vi "Dashboard Main.vi"() -> ()   [LabVIEW 2019]
uses:
  <vilib>/Utility/miscctls.llb/LVRowAndColumnTypeDef.ctl
  <vilib>/event_ctls.llb/eventvkey.ctl
  <vilib>/Rock Robotics/Network Tables/NT Read Numeric Array.vi
  <vilib>/Rock Robotics/Network Tables/NT Read Boolean.vi
  <vilib>/Rock Robotics/WPI/Dashboard/WPI_DashboardLogging Global.vi
panel:
  in  "Camera Settings Right":T1={"Frame Rate"=30, "Compression"=30, "Size"=1, "DB Camera Config"=FALSE} {"Frame Rate" scale=1.0..30.0; "Compression" scale=100.0..-1.0; "Size" items=["640x480", "320x240", "160x120"]}
  in  "Camera Name Right":string(combo)="No Camera Selection"
  out "Camera Perf":string
  in  "Camera Settings":T1={"Frame Rate"=30, "Compression"=30, "Size"=1, "DB Camera Config"=FALSE} {"Frame Rate" scale=1.0..30.0; "Compression" scale=100.0..-1.0; "Size" items=["640x480", "320x240", "160x120"]}
  in  "TCP":refnum<k5>
  in  "Rec Mode":enum32{"Stop", "Record", "Playback"}(radio)
  out "Robot IP":string
  out "Image Message":string="Timeout in Camera Communications"
  in  "Dashboard Tab":T2(tab)=enum."Custom"
  in  "Select Auto":string(combo)="Select Autonomous ..."
  out "NT Connection":bool
  out "MotorChart R":cluster{"Numeric":dbl, "Numeric":dbl}(graph)
  out "MotorChart L":cluster{"Numeric":dbl, "Numeric":dbl}(graph)
  out "MotorSliders R":cluster{"MotorSlide1":dbl, "MotorSlide2":dbl} {"MotorSlide2" scale=-1.0..1.0 scale format="%#_2e"; "MotorSlide1" scale=-1.0..1.0 scale format="%#_2e"}
  out "MotorSliders L":cluster{"MotorSlide1":dbl, "MotorSlide2":dbl} {"MotorSlide2" scale=-1.0..1.0 scale format="%#_2e"; "MotorSlide1" scale=-1.0..1.0 scale format="%#_2e"}
  out "Gyro":dbl(knob) scale=0.0..360.0
  out "JS1 Z":dbl(slide) scale=-1.0..1.0 scale format="%#_2e"
  out "JS1 Graph":cluster{"X":dbl, "Y":dbl}[](graph)
  out "JS1 Buttons":T3
  out "JS2 Z":dbl(slide) scale=-1.0..1.0 scale format="%#_2e"
  out "JS2 Graph":cluster{"X":dbl, "Y":dbl}[](graph)
  out "JS2 Buttons":T3
  out "Mode":T4(ring)=enum."Auto Disabled"
  out "Right Camera Perf":cluster{"Bandwidth (Mbps)":dbl, "FPS":dbl}
  out "Camera Image Right":T5(plugin-control)
  in  "DB/String 9":string
  in  "DB/String 8":string
  in  "DB/String 7":string
  in  "DB/String 6":string
  in  "DB/String 5":string
  in  "DB/String 4":string
  in  "DB/String 3":string
  in  "DB/String 2":string
  in  "DB/String 1":string
  in  "DB/String 0":string
  in  "DB/Slider 0":dbl(slide) scale=0.0..5.0
  in  "DB/Slider 1":dbl(slide) scale=0.0..5.0
  in  "DB/Slider 2":dbl(slide) scale=0.0..5.0
  in  "DB/Slider 3":dbl(slide) scale=0.0..5.0
  out "DB/LED 3":bool
  out "DB/LED 2":bool
  out "DB/LED 1":bool
  out "DB/LED 0":bool
  in  "DB/Button 3":bool
  in  "DB/Button 2":bool
  in  "DB/Button 1":bool
  in  "DB/Button 0":bool caption="New Name"
  out "RET BOOL":bool
  in  "RETICLE":bool caption="RET SHAPE"
  in  "Color":u32(colorbox)=16775210
  out "Intake rotation":dbl(knob) scale=-100.0..100.0
  out "version_note":string
  in  "FIRE PULSE":dbl=0.4 caption="PULSE (s)" min=0.1 max=1.0 step=0.05 format="%#.1g"
  in  "FIRE SPD":dbl=0.4 min=0.4 max=1.0 step=0.1 format="%#.1g"
  out "GAME COLOR":u32(colorbox)
  out "SENSOR COLOR":u32(colorbox)
  out "DRIVER Z":dbl
  out "DRIVER Y":dbl
  out "SHOOTER HT":dbl[](array[slide]) caption="SHOOTER Ht & Spd" scale=0.2..1.0
  out "CW ROTATION":bool
  out "CW DEPLOY":bool
  out "LIFT LOCK":bool
  out "INV DRIVE":bool
  out "FORZA":bool
  out "1 Joystick":bool
  out "NEO MOTOR TEMPS":dbl[](array[slide])=[106.99300699300699] scale=50.0..200.0
  in  "HEIGHT":i32=20
  in  "TOP":i32=130
  in  "WIDE":i32=40
  in  "LEFT":i32=140
  in  "Test Slider":dbl(slide) scale=0.0..100.0 scale format="%#_3g"
  in  "On/Off":bool caption="Solenoid"
  in  "Test Name":u16(ring) items=["Select the test to run..."]
  in  "Test Tree":string(tree)
  in  "Motor":cluster{"Value":dbl, "Enable":bool} {"Value" scale=-1.0..1.0 scale format="%#_3g"}
  out "Progress":T6 {"Test Progress" scale=0.0..100.0}
  in  "Rev/Fwd":cluster{"Forward":bool, "Reverse":bool}
  in  "Test Ring":u16(ring) items=["Monochrome", "Color"]
  out "Cmd Status":string
  in  "Execute Command":bool
  in  "Command Params":string[][](table)
  in  "Command Selection":i32(listbox)
  in  "CheckList":i32(listbox)
  out "Tree":string(tree)
  out "Camera Image":T5(plugin-control)
  out "Background":bool
  in  "Camera Name":string(combo)="No Camera Selection"
  # "HW"
  # "HW"
  # "Joysticks"
  # "Drive Motors"
  # "Front"
  # "Right"
  # "Left"
  # "Back"
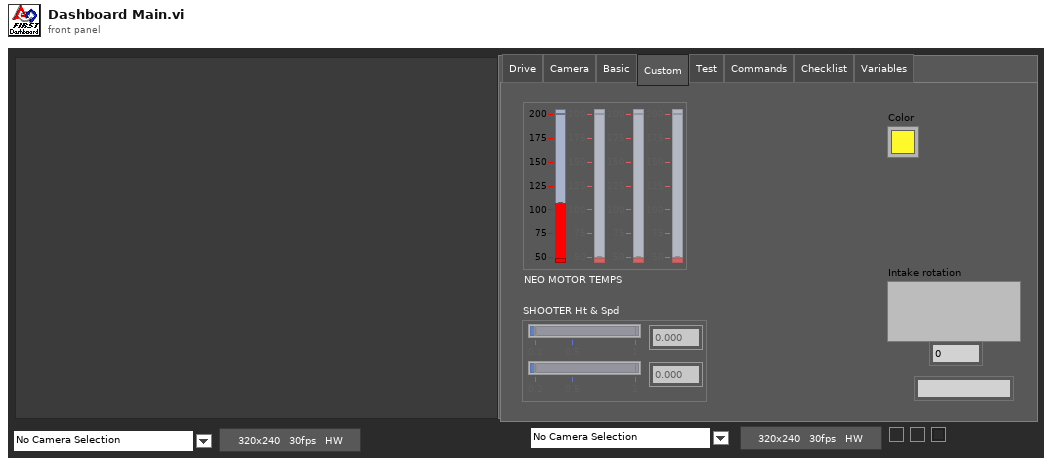
[diagram p1: front panel]
types:
  T1 = cluster{"Frame Rate":i32, "Compression":i32, "Size":u16, "DB Camera Config":bool}
  T2 = enum32{"Drive", "Camera", "Basic", "Custom", "Test", "Commands", "Checklist", "Variables"}
  T3 = cluster{bool, bool, bool, bool, bool, bool, bool, bool, bool, bool, bool, bool}
  T4 = enum8{"Tele-Op Disabled", "Tele-Op Enabled", "Auto Disabled", "Auto Enabled", "Test Disabled", "Test Enabled", "Disconnected", "No Code", "E-Stop"}
  T5 = typedef "IMAQ Image.ctl" = refnum<image>
  T6 = cluster{"Test Progress":u8, "Test Progress Text":string}
  T7 = cluster{"Save Path":path, "Interval (s)":dbl, "Keep":i32}
  T8 = typedef "Image Type" = u32
  T9 = cluster{"IDs":cluster{"RPC field ID":u16, "Unique ID":u16}, "String":string}
  T10 = cluster{"Error Strings":string, "Disable Counts":cluster{u16, u16}, "Rail Faults":cluster{u16, u16, u16}, "Robot IP":string, "DB Mode":u8, "Event Info":cluster{"Name":string, "Type":u8, "Number":u16, "Replay":u8}}
  T11 = cluster{"Storage":cluster{"Disk Free":u64, "RAM Block":u32, "RAM free":u32}, "CPU Utilization":cluster{"CPU % ISR":sgl, "CPU % Time Crit":sgl, "CPU % Timed Str":sgl, "CPU % High":sgl, "CPU % Above":sgl, "CPU % Normal":sgl, "CPU % Low":sgl}, "CAN":cluster{"% Bus Utilization":sgl, "Bus Off Cnt":u32, "TX_FIFO Full Cnt":u32, "Receive Error Cnt":u8, "Transmit Error Cnt":u8}, "HID":cluster{"HID Outputs":u32, "Rumble Low":u16, "Rumble High":u16}[]}
  T12 = cluster{"Status bits":cluster{"Test Mode":bool, "Autonomous":bool, "Enabled":bool, "Code Start":bool, "Brownout":bool, "Reserved 2":bool, "Reserved 3":bool, "E-Stop":bool}, "Code Trace":cluster{"Disabled":bool, "TeleOp":bool, "Auto":bool, "Test":bool}, "Controller Type":enum16{"unknown", "cRIO", "roboRio"}, "Code?":enum16{"unknown", "noCode", "code"}, "Battery V":dbl}
  T13 = cluster{"Control Bits":cluster{"TestMode":bool, "Autonomous":bool, "Enabled":bool, "FMS Present":bool, bool, bool, bool, "E-Stop":bool}, "Team Station ":u8, "Countdown":sgl, "Joystick Values":cluster{"Axes":dbl[], "Buttons":bool[], "POVs":i16[]}[]}
  T14 = cluster{"Axes":dbl[], "Buttons":bool[], "POVs":i16[]}[]
  T15 = cluster{"Axes":dbl[], "Buttons":bool[], "POVs":i16[]}
  T16 = cluster{"Buttons[0]":bool, "Buttons[1]":bool, "Buttons[2]":bool, "Buttons[3]":bool, "Buttons[4]":bool, "Buttons[5]":bool, "Buttons[6]":bool, "Buttons[7]":bool, "Buttons[8]":bool, "Buttons[9]":bool, "Buttons[10]":bool, "Buttons[11]":bool}
  T17 = cluster{"Camera Image":refnum<vi>, "Dashboard Tab":refnum<vi>, "Background":refnum<vi>, "Rec Mode":refnum<vi>, "Test Slider":refnum<vi>, "On/Off ":refnum<vi>, "Test Ring":refnum<vi>, "Rev/Fwd":refnum<vi>, "Test Name":refnum<vi>, "Motor":refnum<vi>, "Progress":refnum<vi>, "CheckList":refnum<vi>, "Tree":refnum<vi>, "Test Tree":refnum<vi>, "Command Params":refnum<vi>, "Command Selection":refnum<vi>, "Execute Command":refnum<vi>, "Cmd Status":refnum<vi>, "Camera Settings":refnum<vi>, "Camera Name":refnum<vi>, "Camera Perf":refnum<vi>, "Camera Settings Right":refnum<vi>, "Camera Name Right":refnum<vi>, "Camera Image Right":refnum<vi>}
  T18 = cluster{"Global Rectangle":i32[], "Contours":cluster{"Contour Type":u32, "ROI Type":u32, "Points":i32[]}[]}
  T19 = cluster{"Left":i32, "Top":i32, "Right":i32, "Bottom":i32}
  T20 = cluster{"Camera Name":string, string, "Saved DB Images Info":cluster{"Save Path":path, "Interval (s)":dbl, "Keep":i32}}
  T21 = cluster{"Camera Name Right":string, string, "Saved DB Images Info":cluster{"Save Path":path, "Interval (s)":dbl, "Keep":i32}}
  T22 = cluster{"Operation":enum16{"Update", "Clear"}, "Color Box":u32}[]
  T23 = typedef "eventvkey.ctl" = enum16{"ASCII", "Enter", "Return", "Shift", "Ctrl", "Alt", "Cmd", "Opt", "Caps", "NumLock", "Clear", "Break", "Up", "Down", "Left", "Right", "Insert", "Delete", "Home", "End", "PageUp", "PageDown", "Escape", "Help", "Pause", "ScrollLock", "F1", "F2", "F3", "F4", "F5", "F6", "F7", "F8", "F9", "F10", "F11", "F12", "F13", "F14", "F15", "F16", "F17", "F18", "F19", "F20", "F21", "F22", "F23", "F24", "Play", "VolumeUp", "VolumeDown", "Mute", "Two Byte Char"}
  T24 = cluster{"Image Size":bool, "Image Type":bool, "Pixel Value":bool, "ROI Information":bool, "Zoom Factor":bool}
  T25 = cluster{"Operation":enum16{"Update", "Clear"}, "Color Box":u32}
  T26 = typedef "LVRowAndColumnTypeDef.ctl" = cluster{"Row":i32, "Column":i32}
  T27 = cluster{"Shift":bool, "Ctrl":bool, "Alt":bool, "Cmd":bool, "Opt":bool}
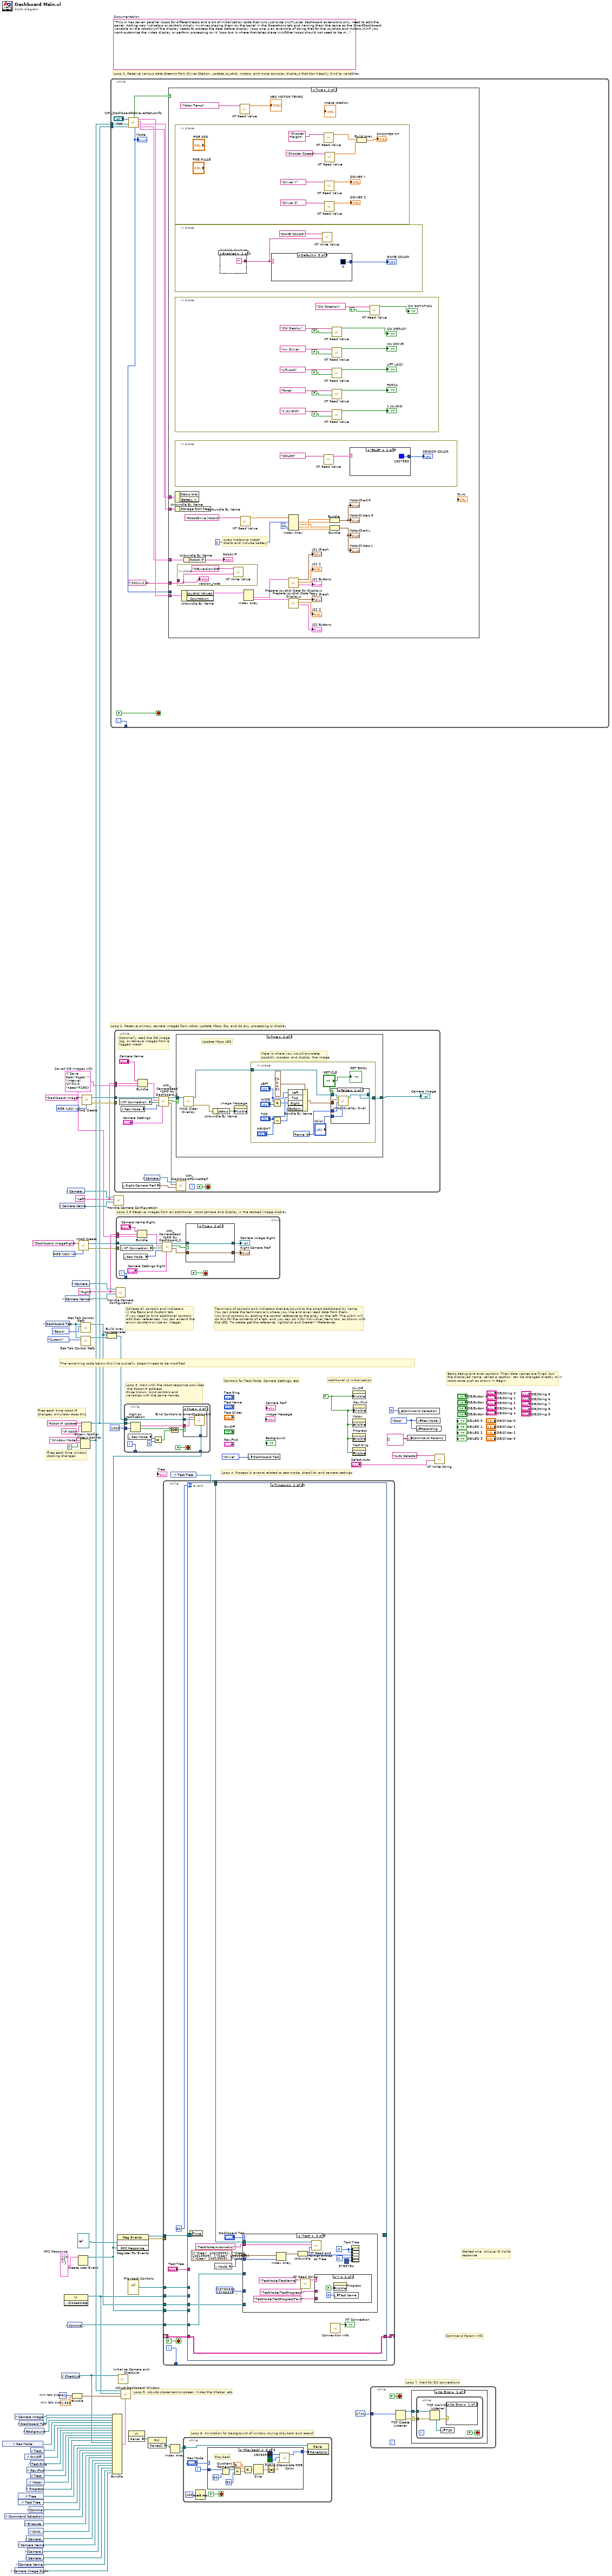
[diagram p0: block diagram]
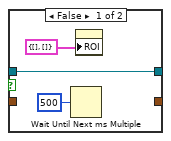
[diagram p2: hidden frame]
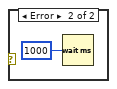
[diagram p3: hidden frame]
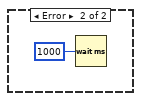
[diagram p4: hidden frame]
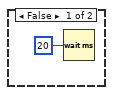
[diagram p5: hidden frame]
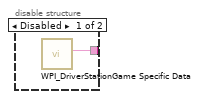
[diagram p6: hidden frame]
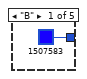
[diagram p7: hidden frame]
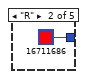
[diagram p8: hidden frame]
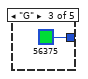
[diagram p9: hidden frame]
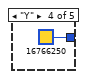
[diagram p10: hidden frame]
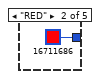
[diagram p11: hidden frame]
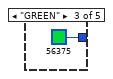
[diagram p12: hidden frame]
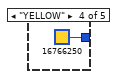
[diagram p13: hidden frame]
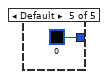
[diagram p14: hidden frame]
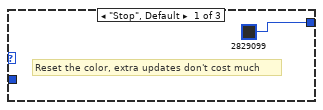
[diagram p15: hidden frame]
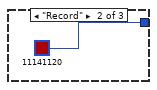
[diagram p16: hidden frame]
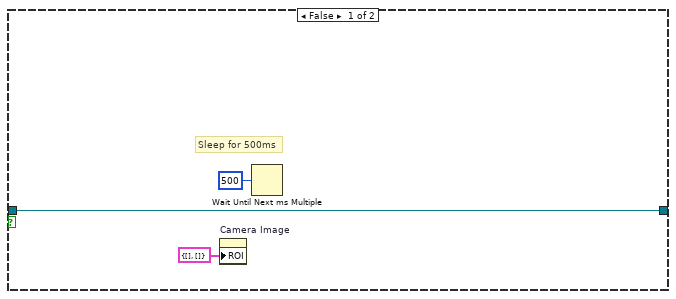
[diagram p18: hidden frame]
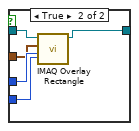
[diagram p19: hidden frame]
diagram:
  w3 = T7 {"Save Path"=path "", "Interval (s)"=1.0, "Keep"=180}  # Saved DB Images Info
  w2 = "Right"
  w1 = "Left"
  w13 = T8 4 items=["Grayscale (U8)", "Grayscale (I16)", "Grayscale (SGL)", "Complex (CSG)", "RGB (U32)", "HSL (U32)", "RGB (U64)"] ("Image Type")
  w29 = T9 {"IDs"={"RPC field ID"=0, "Unique ID"=0}, "String"=""}  # RPC Response
  w52 = 491  # min tab size
  w51 = 1.333  # min tab size
  w59 = enum32{"Stop", "Record", "Playback"}."Stop" ("Rec Mode")
  w36 = FALSE ("Visible")
  (unwired) "This VI has seven parallel loops for different tasks and a bit of initialization code that runs just once.\n\nTypical dashboard extensions only need to edit the panel. Adding new indicators or controls simply involves placing them on the panel in the Operations tab and naming them the same as the SmartDashboard variable on the robot\n\nIf the display needs to process the data before display, loop one is an example of doing that for the joysticks and motors.\n\nIf you want customize the video display or perform processing on it, loop two is where that takes place.\n\nOther loops should not need to be modified. They are pretty standard, and document the task they perform."  # Documentation
  w76 = T8 4 items=["Grayscale (U8)", "Grayscale (I16)", "Grayscale (SGL)", "Complex (CSG)", "RGB (U32)", "HSL (U32)", "RGB (U64)"] ("Image Type")
  # "Loop 2.5 Receive images from an additional  robot camera and display in the tabbed image display"
  # "Command Param Info"
  # "Started one, Unique ID holds\nresponse"
  # "Loop 7. Wait for DS connections"
  # "Basic debug and auto controls: Their data names are fixed, but\nthe displayed name, called a caption, can be changed directly or in\nrobot code such as shown in Begin."
  # "Controls for Test Mode, Camera Settings, etc."
  # "Additional UI Initialization"
  # "Loop 6. Animation for background of window during playback and record"
  # "Fires each time robot IP\nchanges, simulator does this"
  # "Fires each time window\ndocking changes."
  # "Collects all controls and indicators\nin the Basic and Custom tab.\nIf you need to bind additional controls,\nadd their references. You can extend the\nenum constant or use an integer."
  # "The remaining code below this line typically doesn't need to be modified."
  # "Loop 4. Process UI events related to test mode, checklist, and camera settings"
  # "Terminals of controls and indicators that are bound to the smart dashboard by name.\nYou can place the terminals anywhere you like and even read data from them.\nYou bind controls by adding the control reference to the array on the left. The subVI will\ndo this for the contents of a tab, and you can do it for individual items too, as shown with\nthe LED. To create get the reference, right-click and Create>>Reference."
  # "Loop 3. Wait until the robot response provides\n the Robot IP address.\nOnce known, bind controls and\nvariables with the same names."
  # "Loop 5. Adjusts placement onscreen, hides the titlebar, etc."
  # "Loop 1. Receive various data streams from Driver Station, update joystick, motors, and more complex displays that don't easily bind to variables."
  # "Loop 2. Receive primary camera images from robot, update Mbps, fps, and do any processing or display"
  n1 = control-ref of="Rec Mode"() -> (w42:refnum<vi>)
  n2 = control-ref of="Command Selection"() -> (w28:refnum<vi>)
  n3 = control-ref of="Camera Image Right"() -> (w6:refnum<vi>)
  n4 = control-ref of="Camera Image"() -> (w54:refnum<vi>)
  n5 = control-ref of="Tree"() -> (w46:refnum<vi>)
  n6 = control-ref of="Test Tree"() -> (w45:refnum<vi>)
  n7 = control-ref of="Camera Name"() -> (w19:refnum<vi>)
  n8 = control-ref of="Camera Name Right"() -> (w7:refnum<vi>)
  n9 = control-ref of="Dashboard Tab"() -> (w53:refnum<vi>)
  n10 = control-ref of="Execute Command"() -> (w30:refnum<vi>)
  n11 = control-ref of="Background"() -> (w49:refnum<vi>)
  n12 = control-ref of="On/Off"() -> (w40:refnum<vi>)
  n13 = control-ref of="Progress"() -> (w37:refnum<vi>)
  n14 = control-ref of="Camera Settings"() -> (w20:refnum<vi>)
  n15 = control-ref of="Camera Settings Right"() -> (w8:refnum<vi>)
  n16 = control-ref of="Rev/Fwd"() -> (w38:refnum<vi>)
  n17 = control-ref of="Motor"() -> (w43:refnum<vi>)
  n18 = control-ref of="Camera Perf"() -> (w18:refnum<vi>)
  n19 = control-ref of="Cmd Status"() -> (w24:refnum<vi>)
  n20 = control-ref of="Command Params"() -> (w31:refnum<vi>)
  n21 = control-ref of="Test Slider"() -> (w41:refnum<vi>)
  n22 = control-ref of="Test Ring"() -> (w39:refnum<vi>)
  n23 = control-ref of="Test Name"() -> (w44:refnum<vi>)
  n24 = control-ref of="Dashboard Tab"() -> (w57:refnum<vi>)
  n25 = control-ref of="Camera Name"() -> (w21:refnum<vi>)
  n26 = control-ref of="CheckList"() -> (w47:refnum<vi>)
  n27 = property class="VI" props=["Front Panel.Closeable"]() -> (reference out=w58:refnum<vi>)  [unwired: 2 in, 2 out]
  n28 = control-ref of="Camera Name Right"() -> (w9:refnum<vi>)
  n29 = control-ref of="Camera Settings"() -> (w22:refnum<vi>)
  n30 = control-ref of="Command Params"() -> (w23:refnum<vi>)
  n31 = control-ref of="Camera Settings Right"() -> (w10:refnum<vi>)
  n32 = Bundle("min tab size"=w52, "min tab size"=w51) -> (w50:cluster{"min tab size":i32, "min tab size":dbl})  [unwired: 1 in]
  n33 = Create User Event(user event datatype=w29) -> (user event=w25:refnum<user-event>)  [unwired: 1 in, 1 out]
  n34 = call "IMAQ Create"("Image Name"="Dashboard ImageRight", "Image Type"=w13) -> ("New Image"=w12:T5, "error out"=w11:errorcluster)  [unwired: 2 in, 1 out]
  n35 = Obtain Notifier(name (unnamed)="Window Mode", notification data type=TRUE) -> (notifier out=w34:refnum<notifier>)  [unwired: 2 in, 2 out]
  n36 = call <vilib>:"Get Tab Control Refs.vi"("Page Index"=T2."Basic" ("Dashboard Tab"), "TabControl in"=w57) -> ("ControlsOnPage"=w17:refnum<vi>[])  [unwired: 9 in]
  n37 = call <vilib>:"Get Tab Control Refs.vi"("Page Index"=T2."Custom" ("Dashboard Tab"), "TabControl in"=w57) -> ("ControlsOnPage"=w56:refnum<vi>[])  [unwired: 9 in]
  n38 = Obtain Notifier(name (unnamed)="Robot IP Update", notification data type="IP Addr" ("name (unnamed)")) -> (notifier out=w35:refnum<notifier>)  [unwired: 2 in, 2 out]
  n39 = call "IMAQ Create"("Image Name"="Dashboard Image", "Image Type"=w76) -> ("New Image"=w74:T5, "error out"=w73:errorcluster)  [unwired: 2 in, 1 out]
  n40 = Build Array (concatenate)(w17, w56) -> (w55:refnum<vi>[])
  n41 = while {
    tunnel: [w87] -> _
    tunnel: w35 -> [w81]
    tunnel: w34 -> [w78]
    i -> [w87]
    stop <- FALSE stop-if-true
    n42 = call <vilib>:"WPI_DashboardRetrieveStatusInfo.vi"("Binding Refnum"=w81, "Window Mode Notifier"=w78, "TCP Cnx"="TCP") -> ("Power and Errors"=w82:T10, "Robot Metrics"=w85:T11, "Status Info"=w86:T12, "Control Info"=w83:T13, "Robot Mode"=w80:T4, "Process?"=w84:bool)  [unwired: 3 in]
    "Mode" <- w80
    n43 = case shown="True" w84 {
      tunnel: w86 -> [_ w116]
      tunnel: w85 -> [_ w115]
      tunnel: w83 -> [_ w114]
      tunnel: w82 -> [_ w113]
      tunnel: w80 -> [_ _]
      tunnel: "2021v2.0" ("version_note") -> [_ w92]
      frame False {
        n44 = Wait (ms)(milliseconds to wait=u32 20) -> ()  [unwired: 1 out]
      }
      frame True {
        # "swap motors to match\ncharts and include battery"
        n45 = in-place {
          n46 = call-poly <vilib>:"NT Read Value.vi"("Name"="Shooter Height") -> ("Numeric"=w140:dbl)  [unwired: 9 in, 1 out]
          n47 = call-poly <vilib>:"NT Read Value.vi"("Name"="Driver Y") -> ("Numeric"=→"DRIVER Y":dbl)  [unwired: 9 in, 1 out]
          n48 = call-poly <vilib>:"NT Read Value.vi"("Name"="Driver Z") -> ("Numeric"=→"DRIVER Z":dbl)  [unwired: 9 in, 1 out]
          n49 = call-poly <vilib>:"NT Read Value.vi"("Name"="Shooter Speed") -> ("Numeric"=w138:dbl)  [unwired: 9 in, 1 out]
          n50 = Build Array(w140, w138) -> (→"SHOOTER HT":dbl[])
        }
        n51 = in-place {
          n52 = disable-structure shown="Enabled" {
            disable-tunnel: [w122 "" ("Game Specific Data")] -> w119
            frame Disabled {
              n53 = call <vilib>:"WPI_DriverStationGame Specific Data.vi"() -> ("Game Specific Data"=w122:string)  [unwired: 11 in]
            }
            frame Enabled {
            }
          }
          n54 = case shown="Default" w119 {
            tunnel: [u32 1507583 ("SENSOR COLOR") u32 16711686 ("SENSOR COLOR") u32 56375 ("SENSOR COLOR") u32 16766250 ("SENSOR COLOR") u32 0 ("SENSOR COLOR")] -> w121
            frame "B" {
            }
            frame "R" {
            }
            frame "G" {
            }
            frame "Y" {
            }
            frame Default {
            }
          }
          "GAME COLOR" <- w121
          n55 = call-poly <vilib>:"NT Write Value.vi"("String"=w119, "Name"="GAME COLOR") -> ()  [unwired: 9 in, 1 out]
        }
        n56 = in-place {
          n57 = call-poly <vilib>:"NT Read Value.vi"("Default Value"=FALSE, "Name"="CW Deploy") -> ("Boolean"=→"CW DEPLOY":bool)  [unwired: 8 in, 1 out]
          n58 = call-poly <vilib>:"NT Read Value.vi"("Default Value"=FALSE, "Name"="Inv Drive") -> ("Boolean"=→"INV DRIVE":bool)  [unwired: 8 in, 1 out]
          n59 = call-poly <vilib>:"NT Read Value.vi"("Default Value"=FALSE, "Name"="Lift Lock") -> ("Boolean"=→"LIFT LOCK":bool)  [unwired: 8 in, 1 out]
          n60 = call-poly <vilib>:"NT Read Value.vi"("Default Value"=FALSE, "Name"="Forza") -> ("Boolean"=→"FORZA":bool)  [unwired: 8 in, 1 out]
          n61 = call-poly <vilib>:"NT Read Value.vi"("Default Value"=FALSE, "Name"="1 Joystick") -> ("Boolean"=→"1 Joystick":bool)  [unwired: 8 in, 1 out]
          n62 = call-poly <vilib>:"NT Read Value.vi"("Default Value"=FALSE, "Name"="CW Rotation") -> ("Boolean"=→"CW ROTATION":bool)  [unwired: 8 in, 1 out]
        }
        n63 = in-place {
          n64 = call-poly <vilib>:"NT Read Value.vi"("Name"="COLOR") -> ("String"=w130:string)  [unwired: 9 in, 1 out]
          n65 = case shown="\"BLUE\"" w130 {
            tunnel: [u32 1507583 ("SENSOR COLOR") u32 16711686 ("SENSOR COLOR") u32 56375 ("SENSOR COLOR") u32 16766250 ("SENSOR COLOR") u32 0 ("SENSOR COLOR")] -> w129
            frame "BLUE" {
            }
            frame "RED" {
            }
            frame "GREEN" {
            }
            frame "YELLOW" {
            }
            frame Default {
            }
          }
          "SENSOR COLOR" <- w129
        }
        n66 = Unbundle By Name(w116) -> ()  [unwired: 2 out]
        n67 = Unbundle By Name(w115) -> ()  [unwired: 1 out]
        n68 = in-place {
          in-place-border: w92 -> [w117]
          n69 = call-poly <vilib>:"NT Write Value.vi"("String"=w117, "Name"="DB/version/DB") -> ()  [unwired: 9 in, 1 out]
          "version_note" <- w117
        }
        n70 = Unbundle By Name(w114) -> ("Joystick Values"=w104:T14)  [unwired: 1 out]
        n71 = Unbundle By Name(w113) -> ("Robot IP"=→"Robot IP":string)
        n72 = call-poly <vilib>:"NT Read Value.vi"("Name"="Motor Temp") -> ("Numeric Array"=→"NEO MOTOR TEMPS":dbl[])  [unwired: 9 in, 1 out]
        n73 = call-poly <vilib>:"NT Read Value.vi"("Name"="RobotDrive Motors") -> ("Numeric Array"=w94:dbl[])  [unwired: 9 in, 1 out]
        n74 = Index Array(array=w104) -> (element #1=w103:T15, element #2=w99:T15)  [unwired: 2 in]
        n75 = Index Array(array=w94, index #1=1, index #4=0) -> (element #1=w108:dbl, element #2=w109:dbl, element #3=w107:dbl, element #4=w112:dbl)  [unwired: 2 in]
        n76 = call "Prepare Joystick Data for Displays.vi"("Joystick Values"=w103) -> ("Buttons"=→"JS1 Buttons":T16, "Z Axis"=→"JS1 Z":dbl, "Cartesian Data"=→"JS1 Graph":cluster{"X axis":dbl, "X axis":dbl}[])  [unwired: 8 in]
        n77 = call "Prepare Joystick Data for Displays.vi"("Joystick Values"=w99) -> ("Buttons"=→"JS2 Buttons":T16, "Z Axis"=→"JS2 Z":dbl, "Cartesian Data"=→"JS2 Graph":cluster{"X axis":dbl, "X axis":dbl}[])  [unwired: 8 in]
        n78 = Bundle("Numeric"=w107, "Numeric"=w108) -> (→"MotorChart R" →"MotorSliders R":cluster{"Numeric":dbl, "Numeric":dbl})  [unwired: 1 in]
        n79 = Bundle("Numeric"=w109, "Numeric"=w112) -> (→"MotorChart L" →"MotorSliders L":cluster{"Numeric":dbl, "Numeric":dbl})  [unwired: 1 in]
      }
    }
  }
  n80 = Bundle("Camera Image"=w54, "Dashboard Tab"=w53, "Background"=w49, "Rec Mode"=w42, "Test Slider"=w41, "On/Off"=w40, "Test Ring"=w39, "Rev/Fwd"=w38, "Test Name"=w44, "Motor"=w43, "Progress"=w37, "CheckList"=w47, "Tree"=w46, "Test Tree"=w45, "Command Params"=w31, "Command Selection"=w28, "Execute Command"=w30, "Cmd Status"=w24, "Camera Settings"=w20, "Camera Name"=w19, "Camera Perf"=w18, "Camera Settings Right"=w8, "Camera Name Right"=w7, "Camera Image Right"=w6) -> (w48:T17)  [unwired: 1 in]
  n81 = call "Handle Camera Configuration.vi"("CameraNameRef"=w21, "Display Name"=w1, "ClusterRef"=w22) -> ()  [unwired: 9 in]
  n82 = while {
    tunnel: w74 -> [w177]
    tunnel: w73 -> [_]
    tunnel: w3 -> [w170]
    tunnel: w1 -> [w167]
    stop <- FALSE stop-if-true
    # "Optionally read the DB image,\nlog, or retrieve images from a\nlogged match"
    n83 = local read "NT Connection"() -> (w171:bool)
    n84 = local read "Rec Mode"() -> (w174:enum32{"Stop", "Record", "Playback"})
    n85 = local read "Right Camera Perf"() -> (w165:cluster{"Bandwidth (Mbps)":dbl, "FPS":dbl})
    n86 = Bundle("Camera Name"="Camera Name", w167, "Saved DB Images Info"=w170) -> (w169:T20)  [unwired: 1 in]
    n87 = control-ref of="Camera Perf"() -> (w164:refnum<vi>)
    n88 = call <vilib>:"WPI_CameraRead MJPG for Dashboard_2.vi"("Camera Settings"="Camera Settings", "Rec Mode"=w174, "NT Connection"=w171, "Capture Info"=w169, "Image in"=w177) -> ("perf info"=w166:cluster{"Bandwidth (Mbps)":dbl, "fps":dbl}, "Active"=w175:bool, "Image\\ out"=w176:T5)  [unwired: 4 in]
    n89 = case shown="True" w175 {
      tunnel: w176 -> [w180 w184]
      tunnel: [w180 w182] -> w172
      frame False {
        # "Sleep for 500ms"
        n90 = property on="Camera Image" class="ImageControl"("ROI"=T18 {"Global Rectangle"=[], "Contours"=[]}) -> ()  [unwired: 2 in, 2 out]
        n91 = Wait Until Next ms Multiple(millisecond multiple=u32 500) -> ()  [unwired: 1 out]
      }
      frame True {
        # "Here is where you would annotate,\npossibly process, and display the image"
        # "Update Mbps LED"
        n92 = call "IMAQ Clear Overlay"("Image"=w184) -> ("error out"=w185:errorcluster, "Image Out"=w183:T5)  [unwired: 2 in, 7 out]
        n93 = Unbundle By Name(w185) -> ("status"=w186:bool)
        n94 = property on="Image Message" class="Str"("Visible"=w186) -> ()  [unwired: 2 in, 2 out]
        n95 = in-place {
          in-place-border: w183 -> [w199]
          in-place-border: [w198] -> w182
          w197 = u32 0 items=["Frame", "Fill"] ("Drawing Mode (Frame)")
          n96 = Add(x="LEFT", y="WIDE") -> (x+y=w195:i32)
          n97 = Subtract(x="TOP", y="HEIGHT") -> (x-y=w194:i32)
          n98 = Bundle By Name(cluster=T19 {"Left"=0, "Top"=0, "Right"=0, "Bottom"=0} ("Bounding Rectangle"), "Left"="LEFT", "Top"="TOP", "Right"=w195, "Bottom"=w194) -> (w196:T19)
          n99 = case shown="False" "RETICLE" {
            tunnel: w199 -> [w203 w209]
            tunnel: [w204 w208] -> w198
            tunnel: w197 -> [w201 w207]
            tunnel: w196 -> [w202 w206]
            tunnel: "Color" -> [w200 w205]
            frame False {
              n100 = call "IMAQ Overlay Oval"("Color"=w200, "Drawing Mode (Frame)"=w201, "Bounding Rectangle"=w202, "Image"=w203) -> ("Image Out"=w204:T5)  [unwired: 6 in, 1 out]
            }
            frame True {
              n101 = call "IMAQ Overlay Rectangle"("Color"=w205, "Drawing Mode (Frame)"=w207, "Rectangle"=w206, "Image"=w209) -> ("Image Out"=w208:T5)  [unwired: 6 in, 1 out]
            }
          }
          "RET BOOL" <- "RETICLE"
        }
      }
    }
    "Camera Image" <- w172
    n102 = call <vilib>:"WPI_DashboardFormatPerf.vi"("Right Camera Perf"=w165, "Performance"=w166, "String in"=w164) -> ()  [unwired: 9 in]
  }
  n103 = call "Handle Camera Configuration.vi"("CameraNameRef"=w9, "Display Name"=w2, "ClusterRef"=w10) -> ()  [unwired: 9 in]
  n104 = while {
    tunnel: w12 -> [w224]
    tunnel: w11 -> [_]
    tunnel: [w219] -> _
    tunnel: w3 -> [w215]
    tunnel: w2 -> [w212]
    i -> [w219]
    stop <- FALSE stop-if-true
    n105 = local read "NT Connection"() -> (w216:bool)
    n106 = local read "Rec Mode"() -> (w223:enum32{"Stop", "Record", "Playback"})
    n107 = Bundle("Camera Name Right"="Camera Name Right", w212, "Saved DB Images Info"=w215) -> (w214:T21)  [unwired: 1 in]
    n108 = call <vilib>:"WPI_CameraRead MJPG for Dashboard_2.vi"("Camera Settings"="Camera Settings Right", "Rec Mode"=w223, "NT Connection"=w216, "Capture Info"=w214, "Image in"=w224) -> ("perf info"=w210:cluster{"Bandwidth (Mbps)":dbl, "fps":dbl}, "Active"=w218:bool, "Image\\ out"=w221:T5)  [unwired: 4 in]
    n109 = case shown="True" w218 {
      tunnel: w221 -> [w226 w229]
      tunnel: [w226 w229] -> w217
      tunnel: [_ w228] -> w211
      tunnel: w210 -> [_ w228]
      frame False {
        n110 = Wait Until Next ms Multiple(millisecond multiple=u32 500) -> ()  [unwired: 1 out]
        n111 = property on="Camera Image Right" class="ImageControl"("ROI"=T18 {"Global Rectangle"=[], "Contours"=[]}) -> ()  [unwired: 2 in, 2 out]
      }
      frame True {
      }
    }
    "Camera Image Right" <- w217
    "Right Camera Perf" <- w211
  }
  n112 = register-events(refnum<vi> refnum, w25) -> (reference out=w63:refnum<event-registration>, error out=w62:errorcluster)  [unwired: 2 in]
  n113 = call "Initialize Camera and CheckList.vi"("ListBox in"=w47) -> ()  [unwired: 11 in]
  n114 = call "Adjust Dashboard Window.vi"("Sizing Refnums"=w48, "Size Constraints"=w50, "VI"=w58, "WIn Mode"=w34) -> ()  [unwired: 8 in]
  n115 = while {
    tunnel: w55 -> [w241]
    tunnel: w35 -> [w239]
    tunnel: [w237] -> _
    tunnel: u32 1000 ("milliseconds to wait") -> [w236]
    tunnel: w25 -> [w230]
    i -> [w237]
    stop <- FALSE stop-if-true
    n116 = local read "Rec Mode"() -> (w232:enum32{"Stop", "Record", "Playback"})
    n117 = Wait on Notification(notifier=w239, timeout in ms (-1)=w236) -> (notification=w238:string, timed out?=w234:bool)  [unwired: 2 in, 2 out]
    n118 = Equal?(x=w232, y=u16 2 ("Rec Mode")) -> (x = y?=w233:bool)
    n119 = Compound Arithmetic op=OR(invert w234, w233) -> (w235:bool)
    n120 = case shown="True" w235 {
      tunnel: w241 -> [_ w244]
      tunnel: w238 -> [_ w243]
      tunnel: w230 -> [_ w242]
      frame False {
      }
      frame True {
        n121 = call <vilib>:"Bind Controls to SmartDashboard.vi"("RPC ref"=w242, "Bound Control Refs"=w244, "Server IP Address"=w243) -> ()  [unwired: 9 in]
      }
    }
  }
  n122 = vi-ref "Playback Controls.vi"() -> (w64:refnum<vi>)
  n123 = property class="VI"() -> ("Panel"=w66:refnum<vi>)  [unwired: 2 in, 2 out]
  n124 = property class="Pnl"(reference=w66) -> ("Panes[]"=w67:refnum<vi>[])  [unwired: 1 in, 2 out]
  n125 = Index Array(array=w67) -> (element=w65:refnum<vi>)  [unwired: 1 in]
  n126 = control-ref of="Test Tree"() -> (w68:refnum<vi>)
  n127 = while {
    tunnel: [w254] -> _
    tunnel: w68 -> [w253]
    tunnel: w64 -> [w252]
    tunnel: w63 -> [w251]
    tunnel: w62 -> [_]
    tunnel: w58 -> [w250]
    tunnel: w25 -> [w249]
    tunnel: w23 -> [w248]
    shift-right: [w247] -> _
    shift-left: _ -> [w246]
    tunnel: w17 -> [w245]
    i -> [w254]
    stop <- FALSE stop-if-true
    n128 = event shown="[0] Timeout" {
      selector: w251 -> [_ _ _ _ _ _ _ _ _ _ _ _ _ _ _ _ _ _ _ _ _]
      dyn-events: [_ _ _ _ _ _ _ _ _ _ _ _ _ _ _ _ w514 _ _ _ _] -> _
      timeout: u32 60 ("milliseconds to wait") -> [_ _ _ _ _ _ _ _ _ _ _ _ _ _ _ _ _ _ _ _ _]
      tunnel: w253 -> [w266 _ _ _ _ _ _ _ _ _ _ _ _ _ _ _ _ _ _ _ _]
      tunnel: "Test Tree" -> [_ _ _ _ _ _ _ _ _ _ _ w481 w489 w491 w495 w503 _ _ _ _ _]
      tunnel: w252 -> [_ _ _ _ _ _ _ _ _ _ _ _ _ _ _ _ w516 _ w534 _ _]
      tunnel: w250 -> [_ _ _ _ _ _ _ _ _ _ _ _ _ _ _ _ w512 _ _ _ _]
      tunnel: w249 -> [_ _ _ _ _ _ _ _ _ _ _ _ _ _ _ _ w510 _ _ _ _]
      tunnel: w248 -> [w261 _ _ _ _ _ w432 _ _ _ _ _ _ _ _ _ _ _ _ _ _]
      tunnel: [w260 w309 w411 w416 w425 w429 w430 w439 w449 w456 w468 w480 w487 w490 w494 w502 w509 w529 w531 w535 w548] -> w247
      tunnel: w246 -> [w260 w309 w411 w416 w425 w429 w430 _ _ w456 w468 w480 w487 w490 w494 w502 w509 w529 w531 w535 w548]
      tunnel: w245 -> [w258 _ _ _ _ _ _ _ _ _ _ _ _ _ _ _ _ _ _ _ _]
      event Timeout {
        n129 = event-data() -> ()  [unwired: 1 in, 1 out]
        n130 = local read "Mode"() -> (w263:T4)
        n131 = case shown="\"Test\"" "Dashboard Tab" {
          tunnel: w266 -> [_ _ w282 _ _]
          tunnel: "TestMode/Automatic/" ("Name Pattern") -> [_ _ w281 _ _]
          tunnel: T22 [{"Operation"=enum."Clear", "Color Box"=14013909}, {"Operation"=enum."Clear", "Color Box"=14013909}, {"Operation"=enum."Clear", "Color Box"=14013909}, {"Operation"=enum."Clear", "Color Box"=14013909}, {"Operation"=enum."Update", "Color Box"=14013909}, {"Operation"=enum."Update", "Color Box"=16777215}, {"Operation"=enum."Clear", "Color Box"=14013909}, {"Operation"=enum."Clear", "Color Box"=14013909}, {"Operation"=enum."Clear", "Color Box"=14013909}] -> [_ _ w274 _ w302]
          tunnel: w263 -> [_ _ w273 _ w301]
          tunnel: u32[] [15790320, 15790320, 15790320, 15790320, 16777215, 16777215, 15790320, 15790320, 15790320] -> [_ _ _ _ w307]
          tunnel: w261 -> [_ _ _ _ w295]
          tunnel: w258 -> [_ w268 _ _ _]
          frame "Custom", Default {
          }
          frame "Basic" {
            n132 = call <vilib>:"WPI_DashboardUpdateNames.vi"("Controls on Tab"=w268) -> ()  [unwired: 11 in]
          }
          frame "Test" {
            w280 = -2 ("Active Item:Row Number")
            n133 = Index Array(array=w274, index=w273) -> (element=w275:T25)
            n134 = Unbundle(w275) -> ("Operation"=w276:enum16{"Update", "Clear"}, "Color Box"=w277:u32)
            n135 = call <vilib>:"NT Read String.vi"("Name"="TestMode/TestName") -> ("String"=w271:string)  [unwired: 9 in, 1 out]
            n136 = call <vilib>:"NT Read and Format Entries as Tree.vi"("Operation"=w276, "Name Pattern"=w281, "Tree Refnum"=w282) -> ()  [unwired: 7 in, 2 out]
            n137 = case shown="\"\"" w271 {
              tunnel: "TestMode/TestProgress" ("Name") -> [w284 _]
              tunnel: "TestMode/TestProgressText" ("Name") -> [w283 _]
              frame Default {
                n138 = call <vilib>:"NT Read Number.vi"("Name"=w284) -> ("Numeric"=w285:dbl)  [unwired: 9 in, 1 out]
                n139 = call <vilib>:"NT Read String.vi"("Name"=w283) -> ("String"=w286:string)  [unwired: 9 in, 1 out]
                n140 = Bundle("Numeric"=w285, "String"=w286) -> (→"Progress":cluster{"Numeric":dbl, "String":string})  [unwired: 1 in]
              }
              frame "" {
                n141 = property on="Progress" class="Clust (strict)"("Visible"=FALSE) -> ()  [unwired: 2 in, 2 out]
                n142 = local write "Test Name"(u16 0) -> ()
              }
            }
            n143 = property on="Test Tree" class="Tree (strict)"("Active Item Row Number"=w280, "ActiveColNum"=w280, "CellBG"=w277, "Active Item Row Number"=-1 ("Active Item:Row Number"), "CellBG"=u32 5789784 ("Color Box")) -> ()  [unwired: 2 in, 2 out]
          }
          frame "Variables" {
            w292 = string[] ["CameraPublisher", "Usage", "DB"]  # Items to initially close
            n144 = First Call?() -> (First Call?: T/F=w293:bool)
            n145 = control-ref of="Tree"() -> (w294:refnum<vi>)
            n146 = Select(t=w292, s=w293, f=string[] []) -> (s? t:f=w290:string[])
            n147 = call <vilib>:"NT Read and Format Entries as Tree.vi"("Tags to  Close"=w290, "Tree Refnum"=w294) -> ()  [unwired: 8 in, 2 out]
          }
          frame "Commands" {
            w303 = u32 5789784 ("Color Box")
            w304 = T26 {"Row"=-1, "Column"=-2} ("Active Cell:Active Cell")
            w306 = T26 {"Row"=-2, "Column"=-2} ("Active Cell:Active Cell")
            n148 = Index Array(array=w307, index=w301) -> (element=w305:u32)
            n149 = Index Array(array=w302, index=w301) -> (element=w300:T25)
            n150 = Unbundle(w300) -> ("Operation"=w299:enum16{"Update", "Clear"})  [unwired: 1 out]
            n151 = local read "Command Selection"() -> (w298:i32)
            n152 = property on="Command Selection" class="MCListbox (strict)"("ActiveCell"=w306, "CellBG"=w305, "ActiveCell"=w304, "CellBG"=w303) -> ()  [unwired: 2 in, 2 out]
            n153 = call <vilib>:"WPI_DashboardUpdate RPC Info.vi"("Operation"=w299) -> ("update"=w297:bool, "commands"=w296:string[][])  [unwired: 9 in]
            n154 = property on="Command Selection" class="MCListbox (strict)"("ItemNames"=w296) -> ()  [unwired: 2 in, 2 out]
            n155 = property on="Command Params" class="Tbl (strict)"("Active Cell"=w306, "Cell BG Color"=w305, "Active Cell"=w304, "Cell BG Color"=w303) -> ()  [unwired: 2 in, 2 out]
            n156 = call <vilib>:"WPI_DashboardUpdate Command Params.vi"("Update"=w297, "NewVal"=w298, "Commands"=w296, "Param Tbl"=w295) -> ()  [unwired: 7 in, 1 out]
          }
        }
        n157 = call <vilib>:"Connextion Info.vi"() -> ("Connected"=→"NT Connection":bool)  [unwired: 10 in, 1 out]
      }
      event "Test Tree": Value Change {
        # "Show appropriate\ncontrols"
        n158 = event-data() -> ("CtlRef"=w312:refnum<vi>, "NewVal"=w310:string)  [unwired: 1 in]
        n159 = call <vilib>:"WPI_UtilitiesGetTreeIOName.vi"("NewVal"=w310, "TreeControl in"=w312) -> ("I/O Name"=w313:string)  [unwired: 9 in]
        n160 = case shown="\"Camera\"" w313 {
          selector: w313 -> [_ w320 _ w342 w351 _]
          tunnel: w310 -> [_ _ w339 w341 _ w358]
          tunnel: cluster{string[]}[] [{["640x480", "320x240", "160x120"]}, {["Auto", "Fixed indoor", "Fixed outdoor 1", "Fixed outdoor 2", "Fixed fluorescent 1", "Fixed fluorescent 2", "Hold current"]}, {["Auto", "Flicker-free 50 Hz", "Flicker-free 60 Hz", "Hold current"]}, {["None", "Prioritize frame rate", "Prioritize image quality"]}, {["Monochrome", "Color"]}] -> [_ _ _ _ _ w357]
          frame Default {
            w315 = FALSE ("Visible")
            w314 = FALSE ("Visible")
            n161 = property on="Motor" class="Clust (strict)"("Visible"=w314) -> ()  [unwired: 2 in, 2 out]
            n162 = property on="Test Ring" class="Ring (strict)"("Visible"=w314) -> ()  [unwired: 2 in, 2 out]
            n163 = property on="Rev/Fwd" class="Clust (strict)"("Visible"=w315) -> ()  [unwired: 2 in, 2 out]
            n164 = property on="On/Off" class="Bool (strict)"("Visible"=w315) -> ()  [unwired: 2 in, 2 out]
            n165 = property on="Test Slider" class="Slide (strict)"("Visible"=w315) -> ()  [unwired: 2 in, 2 out]
          }
          frame "Analog Out", "Motor", "PWM" {
            w321 = FALSE ("Visible")
            n166 = case shown="\"Analog Out\"" w320 {
              tunnel: [1.0 ("Value") -1.0 ("Value") 0.0 ("Value")] -> w319
              tunnel: [255.0 ("Value") 1.0 ("Value") 5.0 ("Value")] -> w318
              tunnel: [128.0 ("Value") 0.0 ("Value") 0.0 ("Value")] -> w317
              tunnel: [64.0 ("Value") 0.5 ("Value") 1.0 ("Value")] -> w316
              frame "PWM" {
              }
              frame "Motor", Default {
              }
              frame "Analog Out" {
              }
            }
            n167 = property on="Motor" class="Clust (strict)"("Visible"=TRUE) -> ()  [unwired: 2 in, 2 out]
            n168 = property on="Value" class="Slide (strict)"("Value"=w317, "Scale.Minimum"=w319, "Scale.Maximum"=w318, "Scale.Increment"=w316) -> ()  [unwired: 2 in, 2 out]
            n169 = property on="On/Off" class="Bool (strict)"("Visible"=w321) -> ()  [unwired: 2 in, 2 out]
            n170 = property on="Test Slider" class="Slide (strict)"("Visible"=w321) -> ()  [unwired: 2 in, 2 out]
            n171 = property on="Test Ring" class="Ring (strict)"("Visible"=w321) -> ()  [unwired: 2 in, 2 out]
            n172 = property on="Rev/Fwd" class="Clust (strict)"("Visible"=w321) -> ()  [unwired: 2 in, 2 out]
          }
          frame "Servo" {
            w337 = FALSE ("Visible")
            n173 = call <vilib>:"NT Read Number.vi"("Name"=w339) -> ("Numeric"=w338:dbl)  [unwired: 9 in, 1 out]
            n174 = property on="Test Slider" class="Slide (strict)"("Visible"=TRUE, "Scale.Maximum"=170.0 ("Scale.Range:Maximum")) -> ()  [unwired: 2 in, 2 out]
            n175 = local write "Test Slider"(w338) -> ()
            n176 = property on="Motor" class="Clust (strict)"("Visible"=w337) -> ()  [unwired: 2 in, 2 out]
            n177 = property on="Rev/Fwd" class="Clust (strict)"("Visible"=w337) -> ()  [unwired: 2 in, 2 out]
            n178 = property on="On/Off" class="Bool (strict)"("Visible"=w337) -> ()  [unwired: 2 in, 2 out]
            n179 = property on="Test Ring" class="Ring (strict)"("Visible"=w337) -> ()  [unwired: 2 in, 2 out]
          }
          frame "Relay", "Solenoid" {
            w340 = FALSE ("Visible")
            n180 = property on="Motor" class="Clust (strict)"("Visible"=w340) -> ()  [unwired: 2 in, 2 out]
            n181 = property on="Test Slider" class="Slide (strict)"("Visible"=w340) -> ()  [unwired: 2 in, 2 out]
            n182 = Search and Replace String(input string=w341, search string="/Value  **", replace string="/Direction") -> (result string=w347:string)  [unwired: 5 in, 3 out]
            n183 = property on="Test Ring" class="Ring (strict)"("Visible"=w340) -> ()  [unwired: 2 in, 2 out]
            n184 = call <vilib>:"NT Read String.vi"("Name"=w347) -> ("String"=w345:string)  [unwired: 9 in, 1 out]
            n185 = Equal?(x="Both directions", y=w345) -> (x = y?=w343:bool)
            n186 = Not(x=w343) -> (.not. x?=w344:bool)
            n187 = property on="Rev/Fwd" class="Clust (strict)"("Visible"=w343) -> ()  [unwired: 2 in, 2 out]
            n188 = property on="On/Off" class="Bool (strict)"("Visible"=w344, "Caption.Text"=w342) -> ()  [unwired: 2 in, 2 out]
          }
          frame "Compressor", "Digital Out" {
            w350 = FALSE ("Visible")
            # "Get direction and finish"
            n189 = property on="Motor" class="Clust (strict)"("Visible"=w350) -> ()  [unwired: 2 in, 2 out]
            n190 = property on="Test Slider" class="Slide (strict)"("Visible"=w350) -> ()  [unwired: 2 in, 2 out]
            n191 = property on="Test Ring" class="Ring (strict)"("Visible"=w350) -> ()  [unwired: 2 in, 2 out]
            n192 = property on="On/Off" class="Bool (strict)"("Visible"=TRUE, "Caption.Text"=w351) -> ()  [unwired: 2 in, 2 out]
            n193 = property on="Rev/Fwd" class="Clust (strict)"("Visible"=FALSE) -> ()  [unwired: 2 in, 2 out]
          }
          frame "Camera" {
            n194 = call <vilib>:"Get Last Path Segment.vi"("String in"=w358) -> ("String out"=w359:string)  [unwired: 10 in]
            n195 = property on="On/Off" class="Bool (strict)"("Visible"=FALSE) -> ()  [unwired: 2 in, 2 out]
            n196 = property on="Motor" class="Clust (strict)"("Visible"=FALSE) -> ()  [unwired: 2 in, 2 out]
            n197 = property on="Rev/Fwd" class="Clust (strict)"("Visible"=FALSE) -> ()  [unwired: 2 in, 2 out]
            n198 = case shown="\"White Balance  **\"" w359 {
              tunnel: w358 -> [w365 w374 w383 w392 w401 _ w407]
              tunnel: w357 -> [w363 w371 w380 w389 w398 _ _]
              frame "Size  **" {
                n199 = Index Array(array=w363) -> (element=w362:cluster{string[]})  [unwired: 1 in]
                n200 = call <vilib>:"NT Read String.vi"("Name"=w365) -> ("String"=w364:string)  [unwired: 9 in, 1 out]
                n201 = Unbundle(w362) -> (w360:string[])
                n202 = Match First String(2:w360, 3:w364) -> (0:w361:i32)  [unwired: 1 out]
                n203 = property on="Test Ring" class="Ring (strict)"("Value"=w361, "Strings []"=w360) -> ()  [unwired: 2 in, 2 out]
                n204 = property on="Test Ring" class="Ring (strict)"("Visible"=TRUE) -> ()  [unwired: 2 in, 2 out]
                n205 = property on="Test Slider" class="Slide (strict)"("Visible"=FALSE) -> ()  [unwired: 2 in, 2 out]
              }
              frame "White Balance  **" {
                n206 = Index Array(array=w371, index=1) -> (element=w372:cluster{string[]})
                n207 = call <vilib>:"NT Read String.vi"("Name"=w374) -> ("String"=w373:string)  [unwired: 9 in, 1 out]
                n208 = Unbundle(w372) -> (w369:string[])
                n209 = Match First String(2:w369, 3:w373) -> (0:w368:i32)  [unwired: 1 out]
                n210 = property on="Test Ring" class="Ring (strict)"("Value"=w368, "Strings []"=w369) -> ()  [unwired: 2 in, 2 out]
                n211 = property on="Test Ring" class="Ring (strict)"("Visible"=TRUE) -> ()  [unwired: 2 in, 2 out]
                n212 = property on="Test Slider" class="Slide (strict)"("Visible"=FALSE) -> ()  [unwired: 2 in, 2 out]
              }
              frame "Exposure  **" {
                n213 = Index Array(array=w380, index=2) -> (element=w381:cluster{string[]})
                n214 = call <vilib>:"NT Read String.vi"("Name"=w383) -> ("String"=w382:string)  [unwired: 9 in, 1 out]
                n215 = Unbundle(w381) -> (w377:string[])
                n216 = Match First String(2:w377, 3:w382) -> (0:w378:i32)  [unwired: 1 out]
                n217 = property on="Test Ring" class="Ring (strict)"("Value"=w378, "Strings []"=w377) -> ()  [unwired: 2 in, 2 out]
                n218 = property on="Test Ring" class="Ring (strict)"("Visible"=TRUE) -> ()  [unwired: 2 in, 2 out]
                n219 = property on="Test Slider" class="Slide (strict)"("Visible"=FALSE) -> ()  [unwired: 2 in, 2 out]
              }
              frame "Exposure Priority  **" {
                n220 = Index Array(array=w389, index=3) -> (element=w390:cluster{string[]})
                n221 = call <vilib>:"NT Read String.vi"("Name"=w392) -> ("String"=w391:string)  [unwired: 9 in, 1 out]
                n222 = Unbundle(w390) -> (w386:string[])
                n223 = Match First String(2:w386, 3:w391) -> (0:w387:i32)  [unwired: 1 out]
                n224 = property on="Test Ring" class="Ring (strict)"("Value"=w387, "Strings []"=w386) -> ()  [unwired: 2 in, 2 out]
                n225 = property on="Test Ring" class="Ring (strict)"("Visible"=TRUE) -> ()  [unwired: 2 in, 2 out]
                n226 = property on="Test Slider" class="Slide (strict)"("Visible"=FALSE) -> ()  [unwired: 2 in, 2 out]
              }
              frame "Color Enable  **" {
                n227 = Index Array(array=w398, index=4) -> (element=w399:cluster{string[]})
                n228 = call <vilib>:"NT Read String.vi"("Name"=w401) -> ("String"=w400:string)  [unwired: 9 in, 1 out]
                n229 = Unbundle(w399) -> (w395:string[])
                n230 = Match First String(2:w395, 3:w400) -> (0:w396:i32)  [unwired: 1 out]
                n231 = property on="Test Ring" class="Ring (strict)"("Value"=w396, "Strings []"=w395) -> ()  [unwired: 2 in, 2 out]
                n232 = property on="Test Ring" class="Ring (strict)"("Visible"=TRUE) -> ()  [unwired: 2 in, 2 out]
                n233 = property on="Test Slider" class="Slide (strict)"("Visible"=FALSE) -> ()  [unwired: 2 in, 2 out]
              }
              frame Default {
                n234 = property on="Test Ring" class="Ring (strict)"("Visible"=FALSE) -> ()  [unwired: 2 in, 2 out]
                n235 = property on="Test Slider" class="Slide (strict)"("Visible"=FALSE) -> ()  [unwired: 2 in, 2 out]
              }
              frame "Brightness  **", "Color Level  **", "Compression  **", "FPS  **", "Sharpness  **" {
                n236 = call <vilib>:"NT Read Number.vi"("Name"=w407) -> ("Numeric"=w406:dbl)  [unwired: 9 in, 1 out]
                n237 = local write "Test Slider"(w406) -> ()
                n238 = property on="Test Slider" class="Slide (strict)"("Visible"=TRUE, "Scale.Maximum"=100.0 ("Scale.Range:Maximum")) -> ()  [unwired: 2 in, 2 out]
                n239 = property on="Test Ring" class="Ring (strict)"("Visible"=FALSE) -> ()  [unwired: 2 in, 2 out]
              }
            }
          }
        }
        n240 = property on="Progress" class="Clust (strict)"("Visible"=FALSE) -> ()  [unwired: 2 in, 2 out]
      }
      event "Test Name": Mouse Enter {
        # "Populate the ring with the list of tests"
        n241 = event-data() -> ()  [unwired: 1 in, 1 out]
        n242 = call <vilib>:"NT Read String Array.vi"("Name"="TestMode/TestList") -> ("String Array"=w415:string[])  [unwired: 9 in, 1 out]
        n243 = Build Array (concatenate)("Select the test to run...", w415) -> (w414:string[])
        n244 = property on="Test Name" class="Ring (strict)"("Strings []"=w414) -> ()  [unwired: 2 in, 2 out]
      }
      event "Test Name": Value Change {
        w417 = FALSE ("Visible")
        # "Tell the robot the test name to run"
        n245 = event-data() -> ("NewVal"=w421:u16)  [unwired: 1 in]
        n246 = property on="Test Name" class="Ring (strict)"() -> ("Strings []"=w422:string[])  [unwired: 2 in, 2 out]
        n247 = local write "Progress"(T6 {"Test Progress"=0, "Test Progress Text"=""} ("Progress")) -> ()
        n248 = Index Array(array=w422, index=w421) -> (element=w420:string)
        n249 = call <vilib>:"NT Write String.vi"("String"=w420, "Name"="TestMode/TestName") -> ()  [unwired: 9 in, 1 out]
        n250 = property on="Progress" class="Clust (strict)"("Visible"=TRUE) -> ()  [unwired: 2 in, 2 out]
        n251 = property on="Motor" class="Clust (strict)"("Visible"=w417) -> ()  [unwired: 2 in, 2 out]
        n252 = property on="Test Slider" class="Slide (strict)"("Visible"=w417) -> ()  [unwired: 2 in, 2 out]
        n253 = property on="On/Off" class="Bool (strict)"("Visible"=w417) -> ()  [unwired: 2 in, 2 out]
        n254 = property on="Rev/Fwd" class="Clust (strict)"("Visible"=w417) -> ()  [unwired: 2 in, 2 out]
        n255 = property on="Test Ring" class="Ring (strict)"("Visible"=w417) -> ()  [unwired: 2 in, 2 out]
      }
      event "Select Auto": Mouse Enter {
        # "Populate the combo box with the list of autonomous options"
        n256 = event-data() -> ()  [unwired: 1 in, 1 out]
        n257 = call <vilib>:"NT Read String Array.vi"("Name"="Auto List") -> ("String Array"=w424:string[])  [unwired: 9 in, 1 out]
        n258 = property on="Select Auto" class="CmbBox"("Strings[]"=w424) -> ()  [unwired: 2 in, 2 out]
      }
      event "Select Auto": Value Change {
        # "User modified the Auto Selection. Write to NT variable so robot knows."
        n259 = event-data() -> ("NewVal"=w427:string)  [unwired: 1 in]
        n260 = call <vilib>:"NT Write String.vi"("String"=w427, "Name"="Auto Selector") -> ()  [unwired: 9 in, 1 out]
      }
      event "Command Selection": Value Change {
        # "Get the params and show in table"
        n261 = event-data() -> ("NewVal"=w433:i32)  [unwired: 1 in]
        n262 = property on="Command Selection" class="MCListbox (strict)"() -> ("ItemNames"=w431:string[][])  [unwired: 2 in, 2 out]
        n263 = call <vilib>:"WPI_DashboardUpdate Command Params.vi"("NewVal"=w433, "Commands"=w431, "Param Tbl"=w432) -> ()  [unwired: 8 in, 1 out]
      }
      event "Execute Command": Value Change {
        # "Started one, Unique ID holds\nresponse"
        n264 = event-data() -> ()  [unwired: 1 in, 1 out]
        n265 = property on="Command Selection" class="MCListbox (strict)"() -> ("ItemNames"=w444:string[][])  [unwired: 2 in, 2 out]
        n266 = Index Array(array=w444, index (row)="Command Selection", index (col)=0) -> (element=w442:string)
        n267 = call <vilib>:"Invoke Commands.vi"("Command Params"="Command Params", "Function Name"=w442) -> ("Params"=w438:u8, "Started"=w437:bool)  [unwired: 7 in, 1 out]
        n268 = Array Subset(array="Command Params", length (row)=w438) -> (w439:string[][])  [unwired: 3 in]
        n269 = Select(t="Executing" ("Cmd Status"), s=w437, f="" ("Cmd Status")) -> (s? t:f=→"Cmd Status":string)
      }
      event "Command Selection": Double Click {
        n270 = event-data() -> ("Row"=w452:i32)  [unwired: 1 in]
        n271 = property on="Command Selection" class="MCListbox (strict)"() -> ("ItemNames"=w455:string[][])  [unwired: 2 in, 2 out]
        n272 = local read "Command Params"() -> (w451:string[][])
        n273 = Index Array(array=w455, index (row)=w452, index (col)=0) -> (element=w453:string)
        n274 = call <vilib>:"Invoke Commands.vi"("Command Params"=w451, "Function Name"=w453) -> ("Params"=w450:u8, "Started"=w445:bool)  [unwired: 7 in, 1 out]
        n275 = Array Subset(array=w451, length (row)=w450) -> (w449:string[][])  [unwired: 3 in]
        n276 = Select(t="Executing" ("Cmd Status"), s=w445, f="" ("Cmd Status")) -> (s? t:f=w446:string)
        n277 = local write "Cmd Status"(w446) -> ()
      }
      event "CheckList": Double Click {
        # "Shift clears all"
        # "Update symbols on the listbox"
        n278 = event-data() -> ("PlatMods.Shift"=w457:bool, "Row"=w459:i32)  [unwired: 1 in]
        n279 = case shown="True" w457 {
          tunnel: w459 -> [w463 _]
          tunnel: 1 -> [w462 _]
          frame False {
            n280 = property on="CheckList" class="LstBox (strict)"() -> ("Item Symbols"=w461:i32[])  [unwired: 2 in, 2 out]
            n281 = Replace Array Subset(array=w461, new element=w462, index=w463) -> (w460:i32[])
            n282 = property on="CheckList" class="LstBox (strict)"("Item Symbols"=w460) -> ()  [unwired: 2 in, 2 out]
          }
          frame True {
            w464 = 0 ("Top Row")
            n283 = property on="CheckList" class="LstBox (strict)"() -> ("Number of Rows"=w466:u32)  [unwired: 2 in, 2 out]
            n284 = Initialize Array(0, w466) -> (w465:i32[])
            n285 = property on="CheckList" class="LstBox (strict)"("Top Row"=w464, "Value"=w464, "Item Symbols"=w465) -> ()  [unwired: 2 in, 2 out]
          }
        }
      }
      event "CheckList": Key Down {
        # "Update symbols on the listbox\nLeft and right keys check and uncheck"
        n286 = event-data() -> ("VKey"=w470:T23)  [unwired: 1 in]
        n287 = case shown="\"Left\", \"Right\"" w470 {
          selector: w470 -> [w475 _]
          tunnel: eventvkey."Left" ("VKey") -> [w473 _]
          frame "Left", "Right" {
            n288 = Equal?(x=w473, y=w475) -> (x = y?=w474:bool)
            n289 = Select(t=0, s=w474, f=1) -> (s? t:f=w476:i32)
            n290 = property on="CheckList" class="LstBox (strict)"() -> ("Item Symbols"=w479:i32[])  [unwired: 2 in, 2 out]
            n291 = Replace Array Subset(array=w479, new element=w476, index="CheckList") -> (w478:i32[])
            n292 = property on="CheckList" class="LstBox (strict)"("Item Symbols"=w478) -> ()  [unwired: 2 in, 2 out]
          }
          frame Default {
          }
        }
      }
      event "Motor.Enable": Value Change {
        # "When the test mode otor enable helper is set, update that\ntree row item's value"
        n293 = event-data() -> ("NewVal"=w485:bool)  [unwired: 1 in]
        n294 = Unbundle("Motor") -> ("Value"=w484:dbl)  [unwired: 1 out]
        n295 = Select(t=w484, s=w485, f=0.0) -> (s? t:f=w482:dbl)
        n296 = call <vilib>:"NT Write Number.vi"("Numeric"=w482, "Name"=w481) -> ()  [unwired: 9 in, 1 out]
      }
      event "Test Slider": Value Change {
        # "When the test mode slider helper is set, update that\ntree row item's value"
        n297 = event-data() -> ("NewVal"=w488:dbl)  [unwired: 1 in]
        n298 = call <vilib>:"NT Write Number.vi"("Numeric"=w488, "Name"=w489) -> ()  [unwired: 9 in, 1 out]
      }
      event "On/Off": Value Change {
        # "When the test mode on/off helper value is set, update that\ntree row item's value"
        n299 = event-data() -> ("NewVal"=w493:bool)  [unwired: 1 in]
        n300 = Boolean To (0,1)(Boolean=w493) -> (0, 1=w492:i16)
        n301 = call <vilib>:"NT Write Number.vi"("Numeric"=w492, "Name"=w491) -> ()  [unwired: 9 in, 1 out]
      }
      event "Rev/Fwd": Value Change {
        # "When the test mode helper value for relays is set, update that\ntree row item's value"
        n302 = event-data() -> ("NewVal.Forward"=w501:bool, "NewVal.Reverse"=w500:bool)  [unwired: 1 in]
        n303 = Boolean To (0,1)(Boolean=w501) -> (0, 1=w497:i16)
        n304 = Boolean To (0,1)(Boolean=w500) -> (0, 1=w499:i16)
        n305 = Negate(x=w499) -> (-x=w498:i16)
        n306 = Add(x=w497, y=w498) -> (x+y=w496:i16)
        n307 = call <vilib>:"NT Write Number.vi"("Numeric"=w496, "Name"=w495) -> ()  [unwired: 9 in, 1 out]
      }
      event "Test Ring": Value Change {
        # "When a test mode helper value is selected from the ring,\nset the tree item's variable to the string value"
        n308 = event-data() -> ("NewVal"=w505:u16)  [unwired: 1 in]
        n309 = property on="Test Ring" class="Ring (strict)"() -> ("Strings []"=w506:string[])  [unwired: 2 in, 2 out]
        n310 = Index Array(array=w506, index=w505) -> (element=w504:string)
        n311 = call <vilib>:"NT Write String.vi"("String"=w504, "Name"=w503) -> ()  [unwired: 9 in, 1 out]
      }
      event "Rec Mode": Value Change {
        # "Update globals for recording mode and path to read log from.\nClear when logging and let NetworkTables set path for vision to\nuse."
        n312 = event-data() -> ("NewVal"=w517:enum32{"Stop", "Record", "Playback"})  [unwired: 1 in]
        n313 = global write "WPI_DashboardLogging Global.vi" "Logging Filename"(path "") -> ()
        n314 = global write "WPI_DashboardLogging Global.vi" "Recording"(w517) -> ()
        n315 = case shown="\"Playback\"" w517 {
          tunnel: w516 -> [_ w519 w528]
          tunnel: [_ _ w527] -> w514
          tunnel: [_ _ w526] -> _
          tunnel: w512 -> [_ _ w524]
          tunnel: cluster{i32, i32} {-250, 170} -> [_ _ w523]
          tunnel: [_ _ T24 {"Image Size"=TRUE, "Image Type"=TRUE, "Pixel Value"=TRUE, "ROI Information"=TRUE, "Zoom Factor"=FALSE} ("Image Information Shown:All Elements")] -> w507
          tunnel: [_ _ TRUE ("Zoom Factor")] -> w508
          tunnel: w510 -> [_ _ w520]
          frame Default {
          }
          frame "Stop", "Record" {
            # "Place Window too"
            n316 = invoke class="VI" method="FP.Close"(reference=w519) -> (reference out=w518:refnum<vi>)  [unwired: 2 in, 2 out]
            n317 = invoke class="VI" method="Abort VI"(reference=w518) -> ()  [unwired: 2 in, 3 out]
          }
          frame "Playback" {
            n318 = call "Open Playback Panel.vi"("Offset"=w523, "DB VI Ref"=w524, "Playback in"=w528) -> ("Playback out"=w525:refnum<vi>)  [unwired: 8 in]
            n319 = register-events(w525, w520) -> (reference out=w527:refnum<event-registration>, error out=w526:errorcluster)  [unwired: 2 in]
          }
        }
        n320 = property on="Camera Image Right" class="ImageControl"("Image Information Shown"=w507, "Image Information Visible"=w508) -> ()  [unwired: 2 in, 2 out]
        n321 = property on="Camera Image" class="ImageControl"("Image Information Shown"=w507, "Image Information Visible"=w508) -> ()  [unwired: 2 in, 2 out]
        n322 = call <vilib>:"WPI_DashboardNT Log FieldName Cache.vi"("Operation"=enum16{"Lookup/Add", "Index", "Clear"}."Clear") -> ()  [unwired: 8 in, 3 out]
      }
      event Panel Close {
        w530 = enum32{"Stop", "Record", "Playback"}."Stop" ("Rec Mode")
        # "Playback window has been closed, abort"
        n323 = event-data() -> ()  [unwired: 1 in, 4 out]
        n324 = local write "Rec Mode"(w530) -> ()
        n325 = global write "WPI_DashboardLogging Global.vi" "Recording"(w530) -> ()
      }
      event Panel Close {
        # "Abort playback window and ourself"
        n326 = event-data() -> ()  [unwired: 1 in, 4 out]
        n327 = invoke class="VI" method="FP.Close"(reference=w534) -> (reference out=w533:refnum<vi>)  [unwired: 2 in, 2 out]
        n328 = invoke class="VI" method="Abort VI"(reference=w533) -> (error out=w532:errorcluster)  [unwired: 2 in, 2 out]
        n329 = invoke class="VI" method="Abort VI"(error in=w532) -> ()  [unwired: 2 in, 3 out]
      }
      event User Event {
        n330 = event-data() -> ("IDs"=w541:cluster{"RPC field ID":u16, "Unique ID":u16}, "String"=w540:string)  [unwired: 1 in]
        n331 = Bundle("IDs"=w541, "String"=w540) -> (w539:T9)  [unwired: 1 in]
        n332 = call <vilib>:"Retrieve RPC Response.vi"("RPC Response"=w539) -> ("Output"=w537:string[][])  [unwired: 10 in]
        n333 = Build Array (concatenate)(w535, w537) -> (w536:string[][])
        n334 = local write "Command Params"(w536) -> ()
        n335 = local write "Cmd Status"("" ("Cmd Status")) -> ()
      }
      event "Tree": Double Click {
        n336 = event-data() -> ("PlatMods"=w547:T27, "Tag"=w544:string)  [unwired: 1 in]
        n337 = Unbundle(w547) -> ("Shift"=w546:bool)  [unwired: 4 out]
        n338 = String Subset(string=w544, length (rest)=1 ("length (rest)")) -> (substring=w543:string)  [unwired: 1 in]
        n339 = Not(x=w546) -> (.not. x?=w545:bool)
        n340 = case shown="\"/\"" w543 {
          tunnel: w544 -> [_ w550]
          tunnel: w545 -> [_ w549]
          frame Default {
          }
          frame "/" {
            n341 = call <vilib>:"NT Update Persistence.vi"("Persistence"=w549, "Name"=w550) -> ()  [unwired: 9 in, 1 out]
          }
        }
      }
    }
  }
  n342 = while {
    tunnel: w65 -> [w552]
    i -> [w555]
    stop <- FALSE stop-if-true
    n343 = Wait (ms)(milliseconds to wait=u32 100) -> ()  [unwired: 1 out]
    n344 = case shown="\"Playback\"" "Rec Mode" {
      tunnel: w555 -> [_ _ w570]
      tunnel: [u32 2829099 ("Base Color") u32 11141120 ("Target Color") w559] -> w551
      frame "Stop", Default {
        # "Reset the color, extra updates don't cost much"
      }
      frame "Record" {
      }
      frame "Playback" {
        # "Playback"
        n345 = Quotient & Remainder(x=w570, y=u32 50 ("milliseconds to wait")) -> (x-y*floor(x/y)=w566:u32)  [unwired: 1 out]
        n346 = Divide(x=w566, y=u32 50 ("milliseconds to wait")) -> (x/y=w563:dbl)
        n347 = Multiply(x=6.283185307179586, y=w563) -> (x*y=w568:dbl)
        n348 = Sine(x=w568) -> (sin(x)=w567:dbl)
        n349 = Absolute Value(x=w567) -> (abs(x)=w560:dbl)
        n350 = call "Interpolate RGB Color.vi"("Proportion"=w560, "Target Color"=u32 30976, "Base Color"=u32 2829099) -> ("Result Color"=w559:u32)  [unwired: 8 in]
      }
    }
    n351 = property class="Pane"(reference=w552, "PaneColor"=w551) -> ()  [unwired: 1 in, 2 out]
  }
  n352 = local write "Dashboard Tab"(T2."Drive" ("Dashboard Tab")) -> ()
  n353 = property on="On/Off" class="Bool (strict)"("Visible"=w36) -> ()  [unwired: 2 in, 2 out]
  n354 = property on="Motor" class="Clust (strict)"("Visible"=w36) -> ()  [unwired: 2 in, 2 out]
  n355 = property on="Progress" class="Clust (strict)"("Visible"=w36) -> ()  [unwired: 2 in, 2 out]
  n356 = property on="Test Ring" class="Ring (strict)"("Visible"=w36) -> ()  [unwired: 2 in, 2 out]
  n357 = property on="Rev/Fwd" class="Clust (strict)"("Visible"=w36) -> ()  [unwired: 2 in, 2 out]
  n358 = while {
    tunnel: u16 1741 ("timeout ms (25000)") -> [w572]
    stop <- FALSE stop-if-true
    n359 = TCP Create Listener(10:w572) -> (0:w571:errorcluster, 3:w573:refnum<k5>)  [unwired: 4 in, 1 out]
    n360 = case shown="No Error" w571 {
      selector: w571 -> [w575 _]
      tunnel: w573 -> [w576 _]
      frame No Error {
        n361 = while {
          tunnel: w576 -> [w579]
          tunnel: w575 -> [w578]
          stop <- FALSE stop-if-true
          n362 = TCP Wait On Listener(8:w578, 11:w579) -> (0:w580:errorcluster, 4:w581:refnum<k5>)  [unwired: 2 in, 3 out]
          n363 = local write "TCP"(w581) -> ()
          n364 = case shown="No Error" w580 {
            frame No Error {
            }
            frame Error {
              n365 = Wait (ms)(milliseconds to wait=u32 1000) -> ()  [unwired: 1 out]
            }
          }
        }
      }
      frame Error {
        n366 = Wait (ms)(milliseconds to wait=u32 1000) -> ()  [unwired: 1 out]
      }
    }
  }
  n367 = local write "Command Selection"(u16 0 ("milliseconds to wait")) -> ()
  n368 = local write "Command Params"(string[][] [] ("Command Params")) -> ()
  n369 = global write "WPI_DashboardLogging Global.vi" "Recording"(w59) -> ()
  n370 = local write "Rec Mode"(w59) -> ()
  n371 = call <vilib>:"NT Write String.vi"("String"="Select Auto", "Name"="Auto Selector") -> ()  [unwired: 9 in, 1 out]
